vi "Get System Parameter.vi"(8 "error in (no error)":errorcluster caption="错误输入（无错误）", 10 "propertyName":string="BytesPersector", 11 "path":string="Win32_DiskDrive") -> (0 "error out":errorcluster caption="错误输出", 3 "propertyValue":string="512")   [LabVIEW 2013, in "ManagementClass.lvclass"]
uses:
  ManagementClass.lvclass
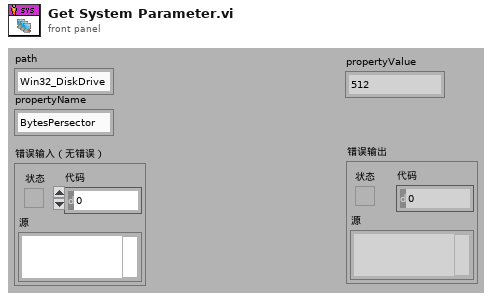
[diagram p1: front panel]
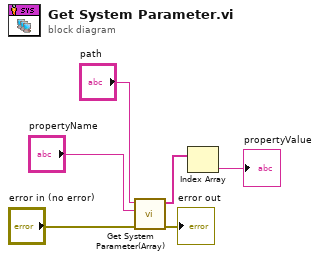
[diagram p0: block diagram]
diagram:
  n1 = call "Get System Parameter(Array).vi"("error in (no error)"="error in (no error)", "propertyName"="propertyName", "path"="path") -> ("error out"=→"error out":errorcluster, "Parameters"=w3:string[])  [unwired: 7 in]
  n2 = Index Array(array=w3) -> (element=→"propertyValue":string)  [unwired: 1 in]
